vi "After Launch Init Core.vi"(8 "error in (no error)":errorcluster, 11 "CS++DMM in":refnum<class "CS++DMM.lvclass">) -> (0 "error out":errorcluster, 3 "CS++DMM out":refnum<class "CS++DMM.lvclass">)   [LabVIEW 2015, in "CS++DMM.lvlib" / "CS++DMM.lvclass"]
doc: "Use <b>Pre Launch init.vi</b> method for sanity checks that are supposed to prevent the actor from launching if they fail. Use <B>this</B> method instead to initialize this actor when it has been activated. A corresponding high priority message will become dispatched before the <B>Actor Core.vi</b> is called.\n\nRefer also to the ongoing discussion at https://decibel.ni.com/content/message/57394#57394."
uses:
  CS++DMM.lvclass
  <vilib>/ActorFramework/Actor/Actor.lvclass
  CS++DMM Messages/Read Single-Point Msg/Read Single-Point Msg.lvclass
  CS++DMM Messages/Read Multi-Point [MP] Msg/Read Multi-Point [MP] Msg.lvclass
  CSPP_Core/Actors/CS++BaseActor/CS++BaseActor.lvclass
  CSPP_Core/Actors/CS++DeviceActor/CS++DeviceActor.lvclass
  CSPP_Core/Classes/CS++ProcessVariables/PVConnection/PVConnection.lvclass
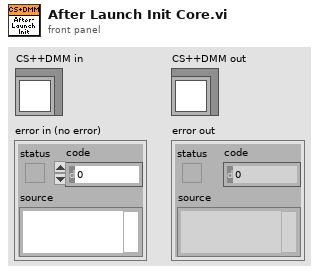
[diagram p1: front panel]
types:
  T1 = cluster{"Read Access":enum8{"Allowed", "Required", "None"}, "Write Access":enum8{"Allowed", "Required", "None"}}
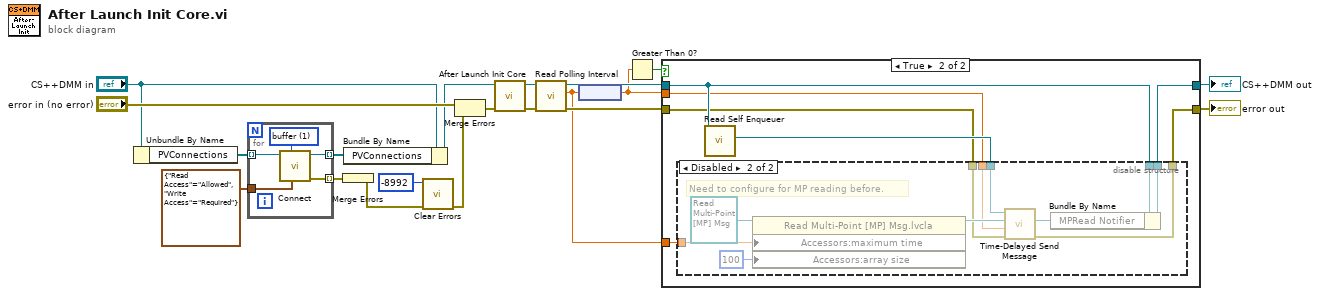
[diagram p0: block diagram]
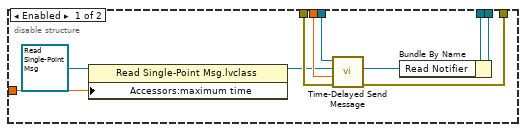
[diagram p3: hidden frame]
diagram:
  n1 = Unbundle By Name("CS++DMM in") -> ("PVConnections"=w7:refnum<class "PVConnection.lvclass">[])
  n2 = for {
    tunnel: w7 -> [w25] mode=indexing
    tunnel: [w24] -> w6 mode=indexing
    tunnel: T1 {"Read Access"=enum."Allowed", "Write Access"=enum."Required"} ("Access (R/W allowed)") -> [w23]
    tunnel: [w22] -> w5 mode=indexing
    w21 = u16 1 items=["commit", "buffer"] ("Mode (commit)")
    n3 = call "Connect.vi"("Access (R/W allowed)"=w23, "Mode (buffer)"=w21, "PVConnection in"=w25) -> ("Error Out"=w22:errorcluster, "PVConnection out"=w24:refnum<class "PVConnection.lvclass">)  [unwired: 7 in]
  }
  n4 = Merge Errors(w5) -> (w2:errorcluster)
  n5 = Bundle By Name(cluster="CS++DMM in", "PVConnections"=w6) -> (w18:refnum<class "CS++DMM.lvclass">)
  n6 = call <vilib>:"Clear Errors.vi"("error in (no error)"=w2, "specific error code to clear (0: all)"=-8992) -> ("error out"=w1:errorcluster)  [unwired: 4 in, 1 out]
  n7 = Merge Errors("error in (no error)", w1) -> (w17:errorcluster)
  n8 = call-parent "After Launch Init Core.vi"("error in (no error)"=w17, "CS++DeviceActor in"=w18) -> ("error out"=w12:errorcluster, "CS++DeviceActor out"=w14:refnum<class "CS++DMM.lvclass">)  [unwired: 8 in]
  n9 = call "Read Polling Interval.vi"("error in (no error)"=w12, "CS++BaseActor in"=w14) -> ("error out"=w11:errorcluster, "Polling Interval"=w8:dbl[unit], "CS++BaseActor out"=w13:refnum<class "CS++DMM.lvclass">)  [unwired: 7 in]
  n10 = node(w8) -> (w10:dbl)
  n11 = Greater Than 0?(x=w10) -> (x > 0?=w9:bool)
  n12 = case shown="True" w9 {
    tunnel: [w27 w34] -> w16
    tunnel: [w26 w28] -> w15
    tunnel: w13 -> [w27 w33]
    tunnel: w11 -> [w26 w31]
    tunnel: w10 -> [_ w30]
    tunnel: w8 -> [_ w29]
    frame False {
    }
    frame True {
      n13 = call <vilib>:"Read Self Enqueuer.vi"("Actor"=w33) -> ("Self Enqueuer"=w32:refnum<class "Message Enqueuer.lvclass">)  [unwired: 10 in]
      n14 = disable-structure shown="Disabled" {
        disable-tunnel: [w44 w47] -> w34
        disable-tunnel: w33 -> [w43 w48]
        disable-tunnel: w32 -> [w41 w51]
        disable-tunnel: w31 -> [w40 w49]
        disable-tunnel: w30 -> [w39 w50]
        disable-tunnel: w29 -> [w36 w52]
        disable-tunnel: [w35 w45] -> w28
        frame Enabled {
          n15 = property class="Read Single-Point Msg.lvclass"(reference=refnum<class "Read Single-Point Msg.lvclass"> refnum ("CS++DMM.lvlib:Read Single-Point Msg.lvclass"), "Accessors:maximum time"=w36) -> (reference out=w37:refnum<class "Read Single-Point Msg.lvclass">)  [unwired: 1 in, 1 out]
          n16 = call <vilib>:"Time-Delayed Send Message.vi"("error in (no error)"=w40, "Milliseconds To Wait"=w39, "Message"=w37, "Message Enqueuer"=w41) -> ("error out"=w35:errorcluster, "Delivery Notifier"=w42:refnum<notifier>)  [unwired: 6 in]
          n17 = Bundle By Name(cluster=w43, "Read Notifier"=w42) -> (w44:refnum<class "CS++DMM.lvclass">)
        }
        frame Disabled {
          # "Need to configure for MP reading before."
          n18 = property class="Read Multi-Point [MP] Msg.lvcla"(reference=refnum<class "Read Multi-Point [MP] Msg.lvclass"> refnum ("CS++DMM.lvlib:Read Multi-Point [MP] Msg.lvclass"), "Accessors:maximum time"=w52, "Accessors:array size"=100 ("array size")) -> (reference out=w54:refnum<class "Read Multi-Point [MP] Msg.lvclass">)  [unwired: 1 in, 1 out]
          n19 = call <vilib>:"Time-Delayed Send Message.vi"("error in (no error)"=w49, "Milliseconds To Wait"=w50, "Message"=w54, "Message Enqueuer"=w51) -> ("error out"=w45:errorcluster, "Delivery Notifier"=w46:refnum<notifier>)  [unwired: 6 in]
          n20 = Bundle By Name(cluster=w48, "MPRead Notifier"=w46) -> (w47:refnum<class "CS++DMM.lvclass">)
        }
      }
    }
  }
  "error out" <- w15
  "CS++DMM out" <- w16
